vi "Server_REPL_Write.vi"(8 "error in (no error)":errorcluster, 9 "Code":string, 11 "Server":path) -> (0 "error out":errorcluster)   [LabVIEW 2020]
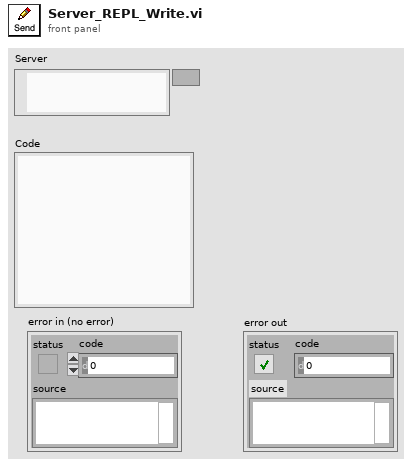
[diagram p1: front panel]
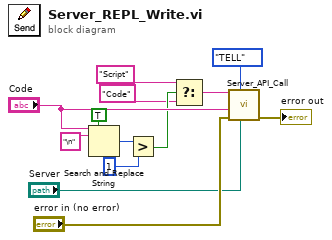
[diagram p0: block diagram]
diagram:
  n1 = Search and Replace String(replace all?=TRUE ("replace all? (F)"), input string="Code", search string="\n" ("replace string (\"\")")) -> (number of replacements=w7:i32)  [unwired: 5 in, 3 out]
  n2 = Greater?(x=w7, y=1) -> (0:w5:bool)
  n3 = Select(t="Script" ("url"), s=w5, f="Code" ("url")) -> (s? t:f=w2:string)
  n4 = call "Server_API_Call.vi"("Server"="Server", "Direction"=enum16{"ASK", "TELL"}."TELL", "error in (no error)"="error in (no error)", "Payload"="Code", "cmd"=w2) -> ("error out"=→"error out":errorcluster)  [unwired: 4 in, 2 out]
